vi "AIARG-MeasureVoltage.vi"() -> ()   [LabVIEW 2018]
uses:
  <vilib>/Analysis/Matrix/Datatypes/RealMatrix.ctl
  <vilib>/Utility/file.llb/Write Delimited Spreadsheet (DBL).vi
  <vilib>/Analysis/Matrix/NI_Matrix.lvlib
panel:
  in  "CSV Path":path
  in  "Output Matrix":T1
  out "D1 Data":dbl[](array[numeric])
  out "SF3 Data":dbl[](array[numeric])
  out "SF2 Data":dbl[](array[numeric])
  out "SF1 Data":dbl[](array[numeric])
  out "L2 Data":dbl[](array[numeric])
  out "L1 Data":dbl[](array[numeric])
  out "Roll Load Data":dbl[](array[numeric])
  out "Pitch Load Data":dbl[](array[numeric])
  out "Yaw Load Data":dbl[](array[numeric])
  out "n Load Data":dbl[](array[numeric])
  out "Axial Load Data":dbl[](array[numeric])
  out "Normal Load Data":dbl[](array[numeric])
  in  "Collect":bool
  in  "Load Roll":dbl
  in  "Load Pitch":dbl
  in  "Load Yaw":dbl
  in  "Load n":dbl
  in  "Load Axial":dbl
  in  "Load Normal":dbl
  out "data":dynamicdata(graph)
  out "SF3":dbl
  out "SF2":dbl
  out "SF1":dbl
  out "D1":dbl
  out "L2":dbl
  out "L1":dbl
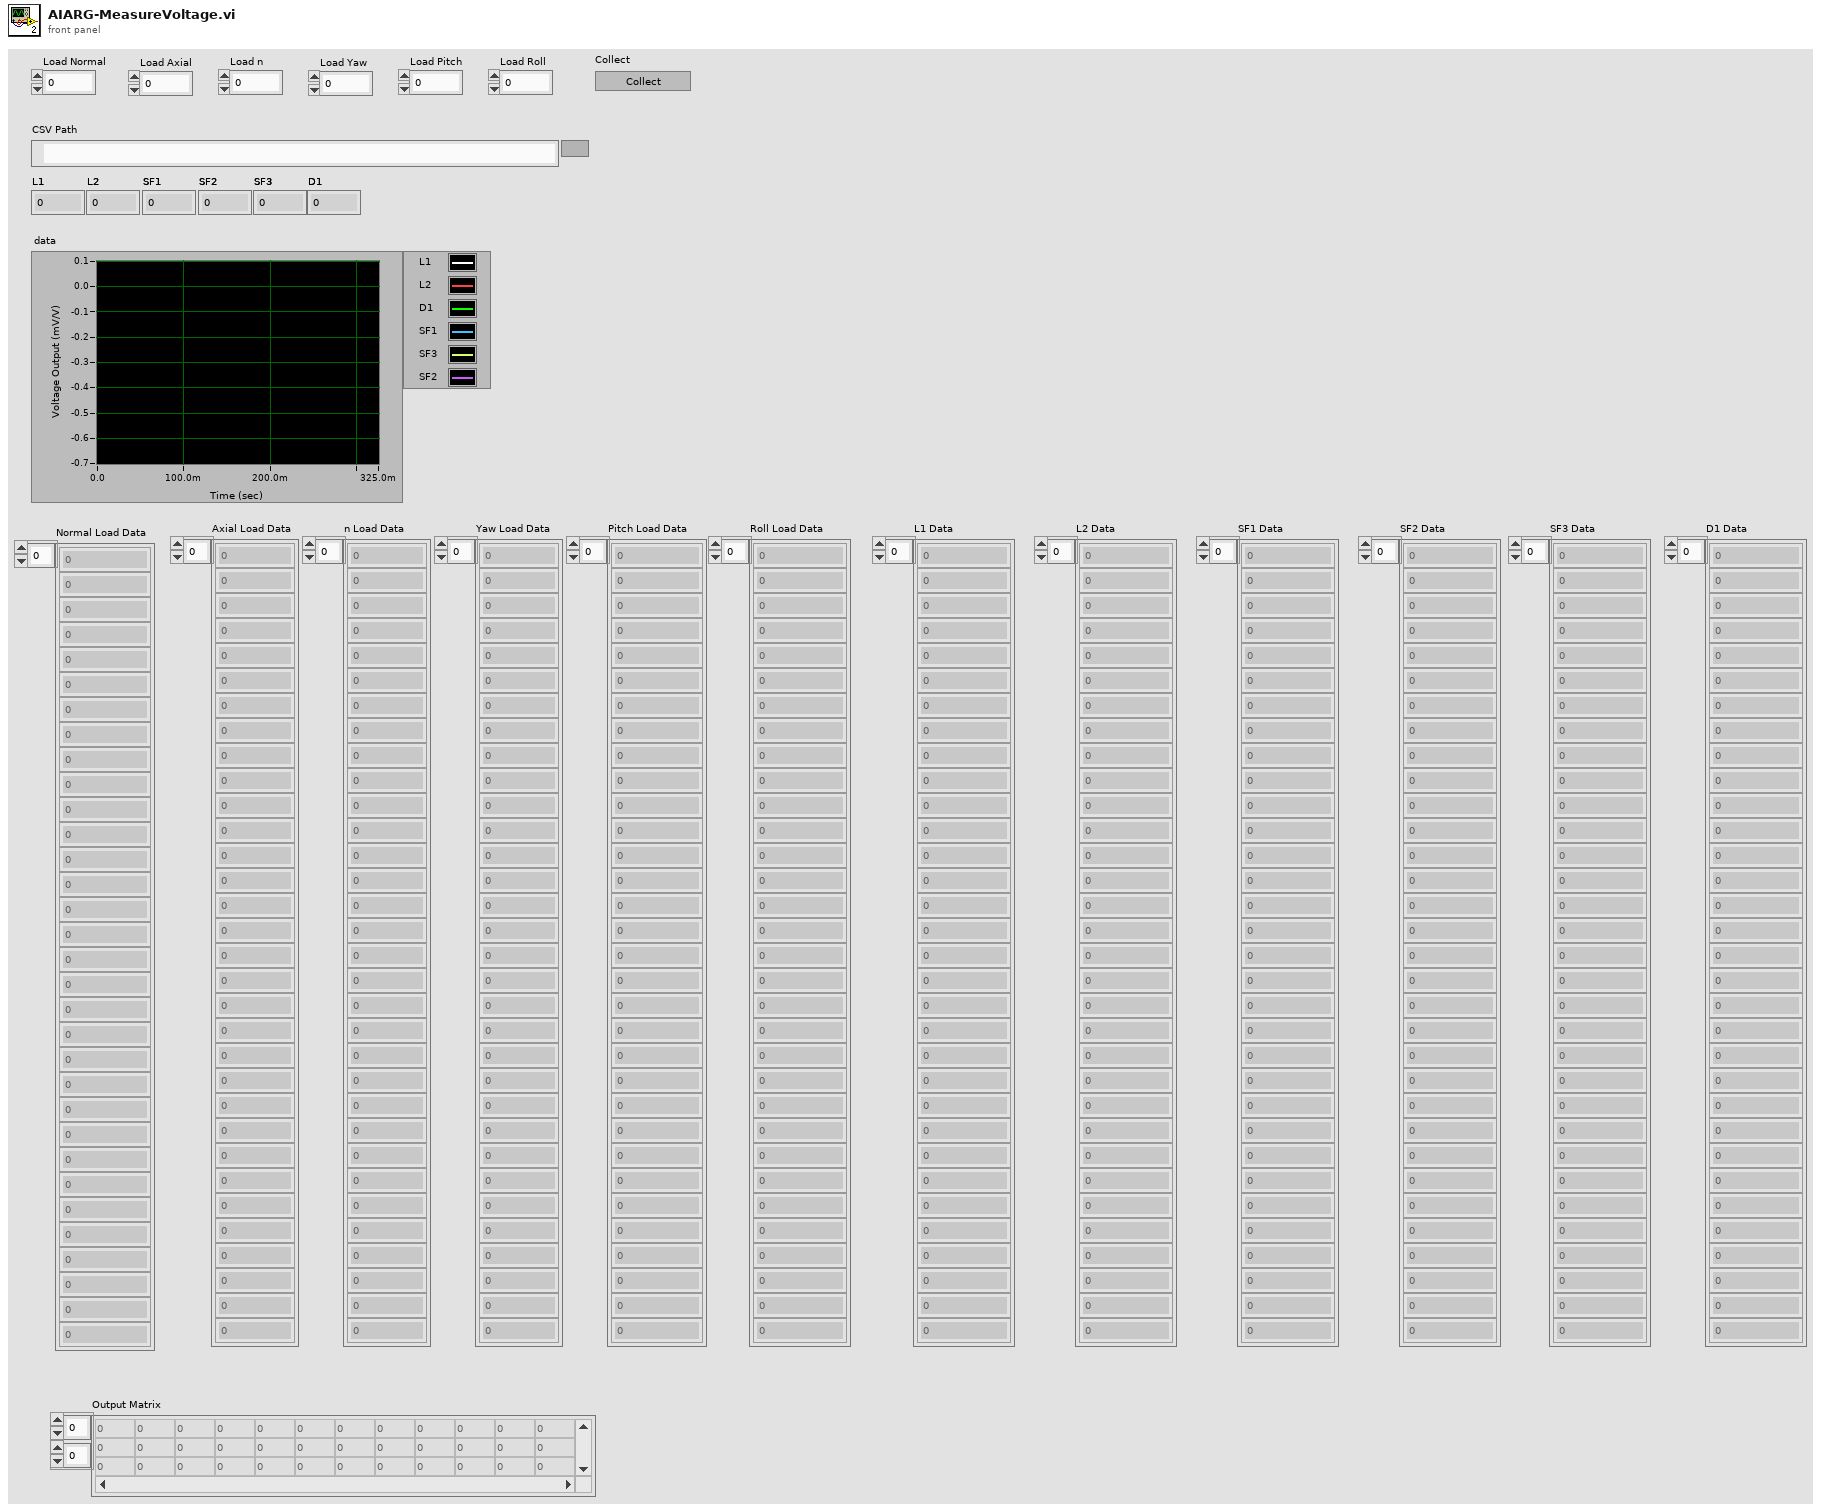
[diagram p1: front panel]
types:
  T1 = typedef "NI_Matrix.lvlib/RealMatrix.ctl" = dbl[][]
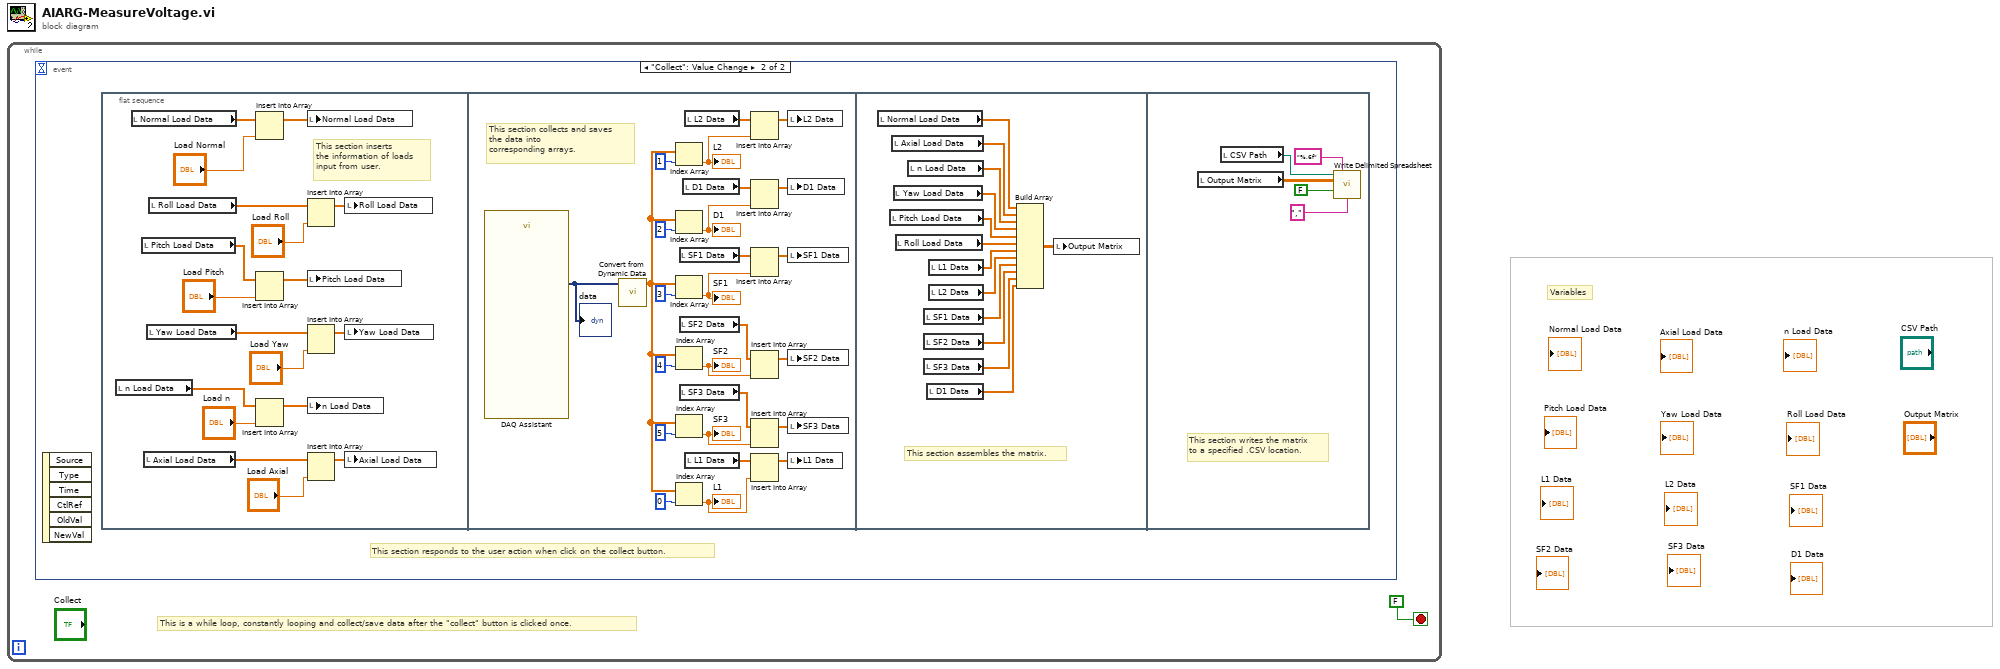
[diagram p0: block diagram]
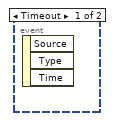
[diagram p2: hidden frame]
diagram:
  # "Variables"
  n1 = while {
    stop <- FALSE stop-if-true
    # "This is a while loop, constantly looping and collect/save data after the \"collect\" button is clicked once."
    n2 = event shown="[1] \"Collect\": Value Change" {
      selector: _ -> [_ _]
      dyn-events: _ -> [_ _]
      timeout: _ -> [_ _]
      event Timeout {
        n3 = event-data() -> ()  [unwired: 1 in, 3 out]
      }
      event "Collect": Value Change {
        # "This section responds to the user action when click on the collect button."
        n4 = event-data() -> ()  [unwired: 1 in, 6 out]
        n5 = flat-sequence {
          frame #0 {
            # "This section inserts\nthe information of loads\ninput from user."
            n6 = local read "n Load Data"() -> (w13:dbl[])
            n7 = local read "Normal Load Data"() -> (w19:dbl[])
            n8 = local read "Pitch Load Data"() -> (w6:dbl[])
            n9 = local read "Axial Load Data"() -> (w16:dbl[])
            n10 = local read "Yaw Load Data"() -> (w9:dbl[])
            n11 = local read "Roll Load Data"() -> (w4:dbl[])
            n12 = Insert Into Array(array=w19, new element="Load Normal") -> (w17:dbl[])  [unwired: 1 in]
            n13 = Insert Into Array(array=w6, new element="Load Pitch") -> (w7:dbl[])  [unwired: 1 in]
            n14 = Insert Into Array(array=w13, new element="Load n") -> (w11:dbl[])  [unwired: 1 in]
            n15 = local write "Normal Load Data"(w17) -> ()
            n16 = Insert Into Array(array=w4, new element="Load Roll") -> (w2:dbl[])  [unwired: 1 in]
            n17 = local write "Pitch Load Data"(w7) -> ()
            n18 = Insert Into Array(array=w9, new element="Load Yaw") -> (w10:dbl[])  [unwired: 1 in]
            n19 = local write "n Load Data"(w11) -> ()
            n20 = Insert Into Array(array=w16, new element="Load Axial") -> (w14:dbl[])  [unwired: 1 in]
            n21 = local write "Roll Load Data"(w2) -> ()
            n22 = local write "Yaw Load Data"(w10) -> ()
            n23 = local write "Axial Load Data"(w14) -> ()
          }
          frame #1 {
            # "This section collects and saves \nthe data into \ncorresponding arrays."
            n24 = call "DAQ Assistant"() -> ("data"=w44:dynamicdata)  [unwired: 17 in, 2 out]
            "data" <- w44
            n25 = call "Convert from Dynamic Data"("Dynamic Data Type"=w44) -> ("Array"=w45:dbl[])  [unwired: 3 in]
            n26 = Index Array(array=w45, index=1) -> (element=w33:dbl)
            "L2" <- w33
            n27 = Index Array(array=w45, index=2) -> (element=w30:dbl)
            "D1" <- w30
            n28 = Index Array(array=w45, index=3) -> (element=w28:dbl)
            "SF1" <- w28
            n29 = Index Array(array=w45, index=4) -> (element=w24:dbl)
            "SF2" <- w24
            n30 = Index Array(array=w45, index=5) -> (element=w21:dbl)
            "SF3" <- w21
            n31 = Index Array(array=w45, index=0) -> (element=w36:dbl)
            "L1" <- w36
            n32 = local read "SF1 Data"() -> (w27:dbl[])
            n33 = local read "SF2 Data"() -> (w25:dbl[])
            n34 = local read "SF3 Data"() -> (w22:dbl[])
            n35 = local read "D1 Data"() -> (w31:dbl[])
            n36 = local read "L2 Data"() -> (w34:dbl[])
            n37 = local read "L1 Data"() -> (w37:dbl[])
            n38 = Insert Into Array(array=w34, new element=w33) -> (w32:dbl[])  [unwired: 1 in]
            n39 = Insert Into Array(array=w31, new element=w30) -> (w29:dbl[])  [unwired: 1 in]
            n40 = Insert Into Array(array=w27, new element=w28) -> (w26:dbl[])  [unwired: 1 in]
            n41 = Insert Into Array(array=w25, new element=w24) -> (w23:dbl[])  [unwired: 1 in]
            n42 = Insert Into Array(array=w22, new element=w21) -> (w20:dbl[])  [unwired: 1 in]
            n43 = Insert Into Array(array=w37, new element=w36) -> (w35:dbl[])  [unwired: 1 in]
            n44 = local write "L2 Data"(w32) -> ()
            n45 = local write "D1 Data"(w29) -> ()
            n46 = local write "SF1 Data"(w26) -> ()
            n47 = local write "SF2 Data"(w23) -> ()
            n48 = local write "SF3 Data"(w20) -> ()
            n49 = local write "L1 Data"(w35) -> ()
          }
          frame #2 {
            # "This section assembles the matrix."
            n50 = local read "Normal Load Data"() -> (w57:dbl[])
            n51 = local read "Pitch Load Data"() -> (w53:dbl[])
            n52 = local read "Axial Load Data"() -> (w56:dbl[])
            n53 = local read "Yaw Load Data"() -> (w54:dbl[])
            n54 = local read "Roll Load Data"() -> (w52:dbl[])
            n55 = local read "n Load Data"() -> (w55:dbl[])
            n56 = local read "SF1 Data"() -> (w49:dbl[])
            n57 = local read "SF2 Data"() -> (w48:dbl[])
            n58 = local read "SF3 Data"() -> (w47:dbl[])
            n59 = local read "D1 Data"() -> (w46:dbl[])
            n60 = local read "L1 Data"() -> (w51:dbl[])
            n61 = local read "L2 Data"() -> (w50:dbl[])
            n62 = Build Array(w57, w56, w55, w54, w53, w52, w51, w50, w49, w48, w47, w46) -> (w58:dbl[][])
            n63 = local write "Output Matrix"(w58) -> ()
          }
          frame #3 {
            # "This section writes the matrix \nto a specified .CSV location."
            n64 = local read "Output Matrix"() -> (w59:T1)
            n65 = local read "CSV Path"() -> (w63:path)
            n66 = call-poly <vilib>:"Write Delimited Spreadsheet.vi"("file path (dialog if empty)"=w63, "format (%.3f)"="%.6f", "2D data"=w59, "append to file? (new file:F)"=FALSE, "delimiter (\\t)"="," ("delimiter (\\t)")) -> ()  [unwired: 9 in, 2 out]
          }
        }
      }
    }
  }
